vi "get single frame.vi"(8 "error in (no error)":errorcluster, 11 "Thorcam in":refnum<class "Thorcam.lvclass">) -> (0 "error out":errorcluster, 3 "Thorcam out":refnum<class "Thorcam.lvclass">)   [LabVIEW 2012, in "Thorcam.lvclass"]
uses:
  Thorcam.lvclass
  Thorcam.lvclass/Thorcam.ctl
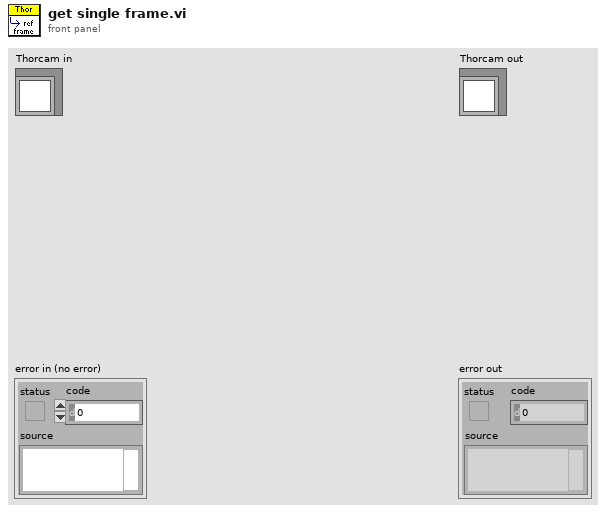
[diagram p1: front panel]
types:
  T1 = typedef "IMAQ Image.ctl" = refnum<image>
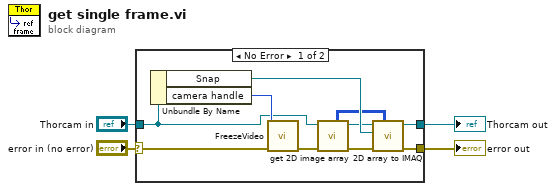
[diagram p0: block diagram]
diagram:
  n1 = case shown="No Error" "error in (no error)" {
    selector: "error in (no error)" -> [w7 w16]
    tunnel: [w6 w16] -> w3
    tunnel: [w5 w15] -> w1
    tunnel: "Thorcam in" -> [w8 w15]
    frame No Error {
      n2 = Unbundle By Name(w8) -> ("Snap"=w14:T1, "camera handle"=w9:u32)
      n3 = call <instrlib>:"FreezeVideo.vi"("error in"=w7, "Camera Handle In"=w9) -> ("error out"=w10:errorcluster)  [unwired: 8 in, 1 out]
      n4 = call-dynamic "get 2D image array.vi"("error in (no error)"=w10, "Thorcam in"=w8) -> ("error out"=w12:errorcluster, "Thorcam out"=w11:refnum<class "Thorcam.lvclass">, "image array out"=w13:u8[][])  [unwired: 7 in]
      n5 = call-dynamic "2D array to IMAQ.vi"("Image Pixels (U8)"=w13, "error in (no error)"=w12, "Image"=w14, "Thorcam in"=w11) -> ("error out"=w6:errorcluster, "Thorcam out"=w5:refnum<class "Thorcam.lvclass">)  [unwired: 6 in]
    }
    frame Error {
    }
  }
  "error out" <- w3
  "Thorcam out" <- w1
